vi "sub_predict-trajectory.vi"(8 "error in":errorcluster, 10 "vy":cluster{"v":dbl, "u":dbl}, 11 "x":dbl[](array[numeric])) -> (0 "error out":errorcluster, 3 "trajectory":dbl[][](array[numeric]))   [LabVIEW 2019]
uses:
  Ctrl/cmd_common.ctl
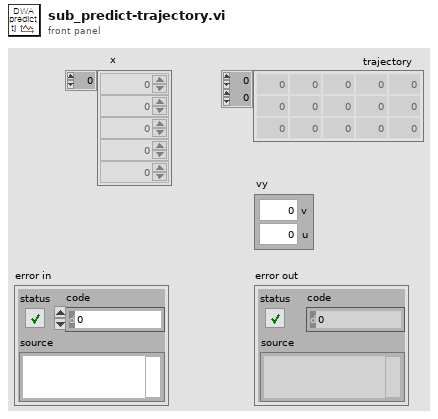
[diagram p1: front panel]
types:
  T1 = typedef "cmd_common.ctl" = enum16{"read", "write"}
  T2 = cluster{"max speed":dbl, "min speed":dbl, "max yaw rate":dbl, "max accel":dbl, "max delta yaw rate":dbl, "v resolution":dbl, "yaw rate resolution":dbl, "dt":dbl, "predict time":dbl, "to goal cost gain":dbl, "speed cost gain":dbl, "obstacle cost gain":dbl, "robot stuck flag cons":dbl, "robot type":enum16{"circle", "rectangle"}, "robot radius":dbl, "robot width":dbl, "robot length":dbl, "obstacles":cluster{"x":dbl, "y":dbl}[], "goal pt":cluster{"x":i32, "y":i32}}
  T3 = cluster{"x":dbl[], "dw":dbl[], "vy":cluster{"v":dbl, "y":dbl}, "trajectory":dbl[][], "best trajectory":dbl[][], "best u":cluster{"v":dbl, "y":dbl}}
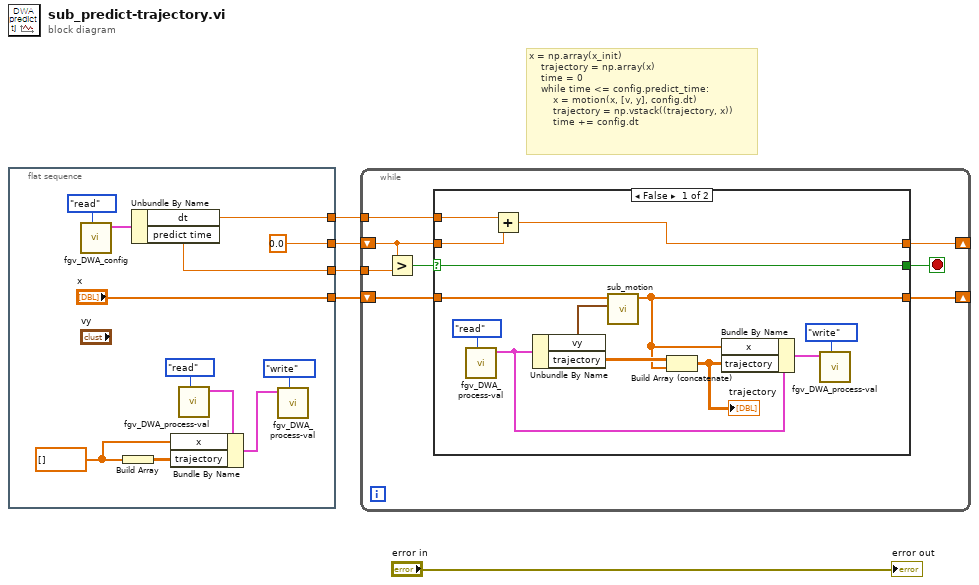
[diagram p0: block diagram]
diagram:
  # "x = np.array(x_init)\n    trajectory = np.array(x)\n    time = 0\n    while time <= config.predict_time:\n        x = motion(x, [v, y], config.dt)\n        trajectory = np.vstack((trajectory, x))\n        time += config.dt"
  n1 = flat-sequence {
    tunnel: [0.0] -> w5
    tunnel: [w14] -> w4
    tunnel: [w13] -> w3
    tunnel: ["x"] -> w1
    frame #0 {
      w6 = dbl[] [] ("x")
      n2 = call "fgv_DWA_config.vi"("cmd"=cmd_common."read") -> ("config out"=w16:T2)  [unwired: 10 in]
      n3 = Build Array(w6) -> (w7:dbl[][])
      n4 = Unbundle By Name(w16) -> ("dt"=w13:dbl, "predict time"=w14:dbl)
      n5 = call "fgv_DWA_process-val.vi"("cmd"=cmd_common."read") -> ("prcess val out"=w8:T3)  [unwired: 10 in]
      n6 = Bundle By Name(cluster=w8, "x"=w6, "trajectory"=w7) -> (w10:T3)
      n7 = call "fgv_DWA_process-val.vi"("cmd"=cmd_common."write", "prcess val"=w10) -> ()  [unwired: 9 in, 1 out]
    }
  }
  n8 = while {
    shift-right: [w20] -> _
    shift-left: w5 -> [w21]
    tunnel: w4 -> [w25]
    tunnel: w3 -> [w22]
    shift-right: [w18] -> _
    shift-left: w1 -> [w19]
    stop <- w23 stop-if-true
    n9 = Greater?(x=w21, y=w25) -> (0:w24:bool)
    n10 = case shown="False" w24 {
      selector: w24 -> [w38 w41]
      tunnel: [w38 w41] -> w23
      tunnel: w22 -> [w37 _]
      tunnel: w21 -> [w36 w40]
      tunnel: [w35 w40] -> w20
      tunnel: w19 -> [w34 w39]
      tunnel: [w26 w39] -> w18
      frame False {
        n11 = call "fgv_DWA_process-val.vi"("cmd"=cmd_common."read") -> ("prcess val out"=w30:T3)  [unwired: 10 in]
        n12 = Add(x=w37, y=w36) -> (x+y=w35:dbl)
        n13 = Unbundle By Name(w30) -> ("vy"=w32:cluster{"v":dbl, "y":dbl}, "trajectory"=w28:dbl[][])
        n14 = call "sub_motion.vi"("vy"=w32, "x"=w34) -> ("x out"=w26:dbl[])  [unwired: 9 in]
        n15 = Build Array (concatenate)(w28, w26) -> (w27:dbl[][])
        "trajectory" <- w27
        n16 = Bundle By Name(cluster=w30, "x"=w26, "trajectory"=w27) -> (w29:T3)
        n17 = call "fgv_DWA_process-val.vi"("cmd"=cmd_common."write", "prcess val"=w29) -> ()  [unwired: 9 in, 1 out]
      }
      frame True {
      }
    }
  }
  "error out" <- "error in"
